vi "onHeartbeat.vi"(8 "error in (no error)":errorcluster, 10 "model in":refnum<class "IModel.lvclass">, 11 "FaultState in":refnum<class "FaultState.lvclass">) -> (0 "error out":errorcluster, 2 "model out":refnum<class "IModel.lvclass">, 3 "FaultState out":refnum<class "FaultState.lvclass">)   [LabVIEW 2016, in "States.lvlib" / "FaultState.lvclass"]
uses:
  FaultState.lvclass
  IModel/IModel.lvclass
  ts_sallv_sedspectrometer/DataTypes/logevent_SummaryState.ctl
  ts_sallv_sedspectrometer/DataTypes/logevent_DetailedState.ctl
  ts_sallv_sedspectrometer/SALLV_sedSpectrometer.lvlib
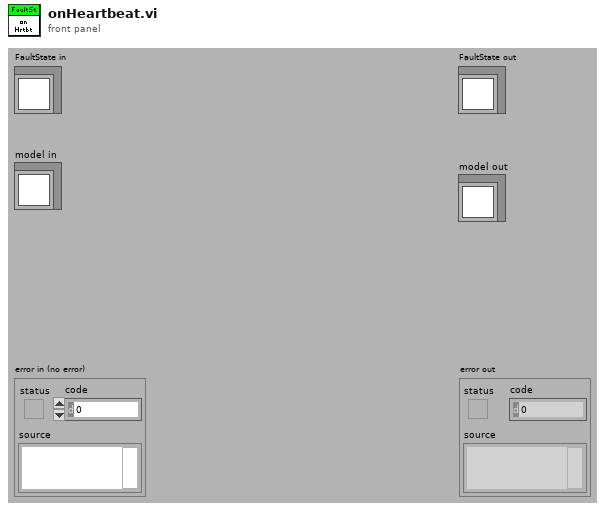
[diagram p1: front panel]
types:
  T1 = typedef "SALLV_sedSpectrometer.lvlib/logevent_DetailedState.ctl" = cluster{"detailedState":enum16{"", "DisabledState", "EnabledState", "FaultState", "OfflineState", "StandbyState"}, "priority":i32}
  T2 = typedef "SALLV_sedSpectrometer.lvlib/logevent_SummaryState.ctl" = cluster{"summaryState":enum16{"", "DisabledState", "EnabledState", "FaultState", "OfflineState", "StandbyState"}, "priority":i32}
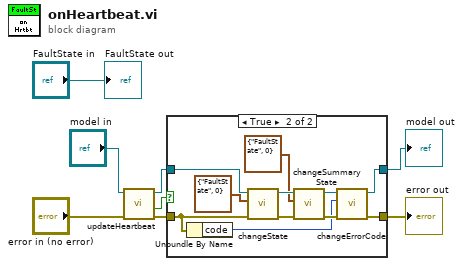
[diagram p0: block diagram]
diagram:
  n1 = call-dynamic "updateHeartbeat.vi"("error in (no error)"="error in (no error)", "IModel in"="model in") -> ("error out"=w3:errorcluster, "resendState?"=w5:bool, "IModel out"=w2:refnum<class "IModel.lvclass">)  [unwired: 7 in]
  n2 = case shown="True" w5 {
    tunnel: [w9 w16] -> w4
    tunnel: w3 -> [w9 w15]
    tunnel: w2 -> [w10 w14]
    tunnel: [w10 w13] -> w1
    frame False {
    }
    frame True {
      n3 = Unbundle By Name(w15) -> ("code"=w17:i32)
      n4 = call-dynamic "changeState.vi"("error in (no error)"=w15, "DetailedState"=T1 {"detailedState"=enum."FaultState", "priority"=0} ("logevent_DetailedState"), "IModel in"=w14) -> ("error out"=w19:errorcluster, "IModel out"=w21:refnum<class "IModel.lvclass">)  [unwired: 7 in]
      n5 = call-dynamic "changeSummaryState.vi"("error in (no error)"=w19, "logevent_SummaryState"=T2 {"summaryState"=enum."FaultState", "priority"=0}, "IModel in"=w21) -> ("error out"=w18:errorcluster, "IModel out"=w20:refnum<class "IModel.lvclass">)  [unwired: 7 in]
      n6 = call-dynamic "changeErrorCode.vi"("error in (no error)"=w18, "error.code"=w17, "IModel in"=w20) -> ("error out"=w16:errorcluster, "IModel out"=w13:refnum<class "IModel.lvclass">)  [unwired: 7 in]
    }
  }
  "error out" <- w4
  "model out" <- w1
  "FaultState out" <- "FaultState in"
